vi "rampa_lab1.vi"() -> ()   [LabVIEW 2025]
uses:
  <vilib>/Utility/file.llb/Write Delimited Spreadsheet (DBL).vi
panel:
  out "Waveform Chart":dynamicdata(graph)
  out "Rpm":dbl
  in  "stop (F)":bool
  # "Velocidad [RPM]"
  # "DETENER"
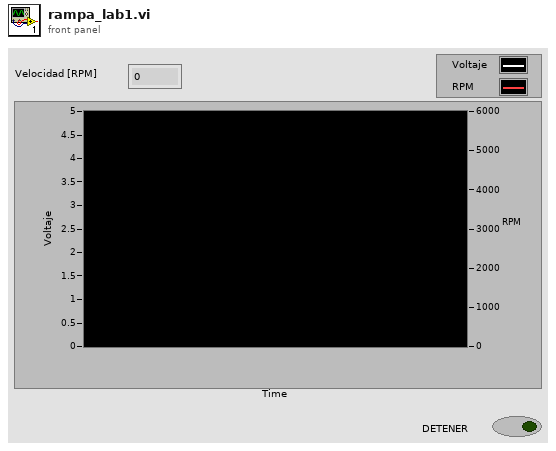
[diagram p1: front panel]
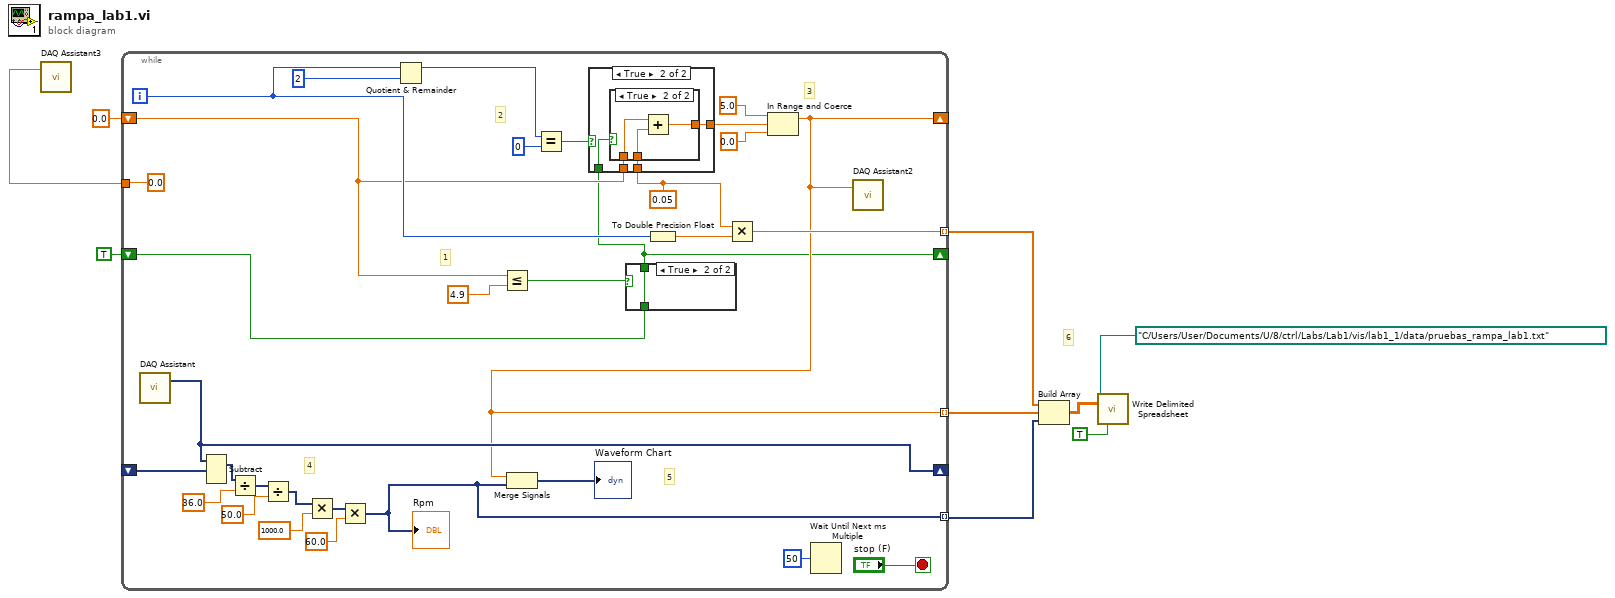
[diagram p0: block diagram]
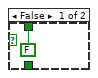
[diagram p2: hidden frame]
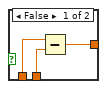
[diagram p4: hidden frame]
diagram:
  # "6"
  n1 = while {
    shift-right: [w39] -> _
    shift-left: _ -> [w38]
    tunnel: [0.0 ("data")] -> w9
    tunnel: [w18] -> w8 mode=indexing
    tunnel: [w27] -> w7 mode=indexing
    tunnel: [w26] -> w6 mode=indexing
    shift-right: [w18] -> _
    shift-left: 0.0 ("x") -> [w15]
    shift-right: [w14] -> _
    shift-left: TRUE -> [w16]
    i -> [w25]
    stop <- "stop (F)" stop-if-true
    w10 = 0.05 ("y")
    # "5"
    # "4"
    # "3"
    # "2"
    # "1"
    n2 = call "DAQ Assistant"() -> ("data"=w39:dynamicdata)  [unwired: 16 in, 3 out]
    n3 = Subtract(1:w38, 2:w39) -> (0:w31:dynamicdata)  [unwired: 1 in, 1 out]
    n4 = Divide(x=w31, y=36.0) -> (x/y=w29:dynamicdata)
    n5 = Divide(x=w29, y=50.0) -> (x/y=w30:dynamicdata)
    n6 = Multiply(x=w30, y=1000.0) -> (x*y=w36:dynamicdata)
    n7 = Multiply(x=w36, y=60.0) -> (x*y=w27:dynamicdata)
    "Rpm" <- w27
    n8 = Quotient & Remainder(x=w25, y=2) -> (x-y*floor(x/y)=w13:i32)  [unwired: 1 out]
    n9 = Less Or Equal?(x=w15, y=4.9) -> (x <= y?=w17:bool)
    n10 = Equal?(x=w13, y=0) -> (x = y?=w23:bool)
    n11 = case shown="True" w17 {
      tunnel: w16 -> [_ w43]
      tunnel: [FALSE w43] -> w14
      frame False {
      }
      frame True {
      }
    }
    n12 = case shown="True" w23 {
      tunnel: w15 -> [w44 w48]
      tunnel: w10 -> [_ w47]
      tunnel: [w44 w46] -> w22
      tunnel: w14 -> [_ w45]
      frame False {
      }
      frame True {
        n13 = case shown="True" w45 {
          tunnel: w48 -> [w49 w54]
          tunnel: w47 -> [w50 w53]
          tunnel: [w51 w52] -> w46
          frame False {
            n14 = Subtract(x=w49, y=w50) -> (x-y=w51:dbl)
          }
          frame True {
            n15 = Add(x=w54, y=w53) -> (x+y=w52:dbl)
          }
        }
      }
    }
    n16 = To Double Precision Float(number=w25) -> (double precision float=w11:dbl)
    n17 = Multiply(x=w10, y=w11) -> (x*y=w26:dbl)
    n18 = In Range and Coerce(upper limit=5.0, x=w22, lower limit=0.0) -> (coerced(x)=w18:dbl)  [unwired: 1 out]
    n19 = Merge Signals(w18, w27) -> (→"Waveform Chart":dynamicdata)
    n20 = Wait Until Next ms Multiple(millisecond multiple=u32 50) -> ()  [unwired: 1 out]
    n21 = call "DAQ Assistant2"("data"=w18) -> ()  [unwired: 17 in, 2 out]
  }
  n22 = call "DAQ Assistant3"("data"=w9) -> ()  [unwired: 17 in, 2 out]
  n23 = Build Array(w6, w8, w7) -> (w4:dbl[][])
  n24 = call-poly <vilib>:"Write Delimited Spreadsheet.vi"("file path (dialog if empty)"=path "C:/Users/User/Documents/U/8/ctrl/Labs/Lab1/vis/lab1_1/data/pruebas_rampa_lab1.txt", "2D data"=w4, "transpose? (no:F)"=TRUE) -> ()  [unwired: 11 in, 2 out]
